vi "training_node.vi"() -> ()   [LabVIEW 2018]
uses:
  <vilib>/Utility/xml.llb/Read From XML File(string).vi
  <vilib>/Utility/xml.llb/Write to XML File(string).vi
panel:
  in  "Training Data Folder":path
  in  "Initialize Weights?":bool
  in  "Weights XML\n(Select Existing File or Name a New File)":path
  in  "Learning Parameter":dbl
  in  "Expected Output":dbl[](array[numeric])
  out "Output":dbl[](array[numeric])
  # "Neural Network Training Node"
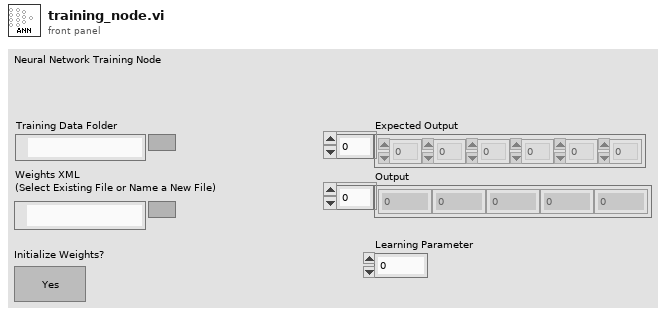
[diagram p1: front panel]
types:
  T1 = cluster{cluster{dbl[][], dbl[][], dbl[][]}, cluster{dbl[], dbl[], dbl[]}}
  T2 = enum16{"open", "replace", "create", "open or create", "replace or create", "replace or create with confirmation"}
  T3 = cluster{"Matrix Product":dbl[], "Matrix Product":dbl[], dbl[]}
  T4 = cluster{cluster{"Updated Weights":dbl[][], "Updated Weights":dbl[][], "Updated Weights":dbl[][]}, cluster{"Updated Biases":dbl[], "Updated Biases":dbl[], "Updated Biases":dbl[]}}
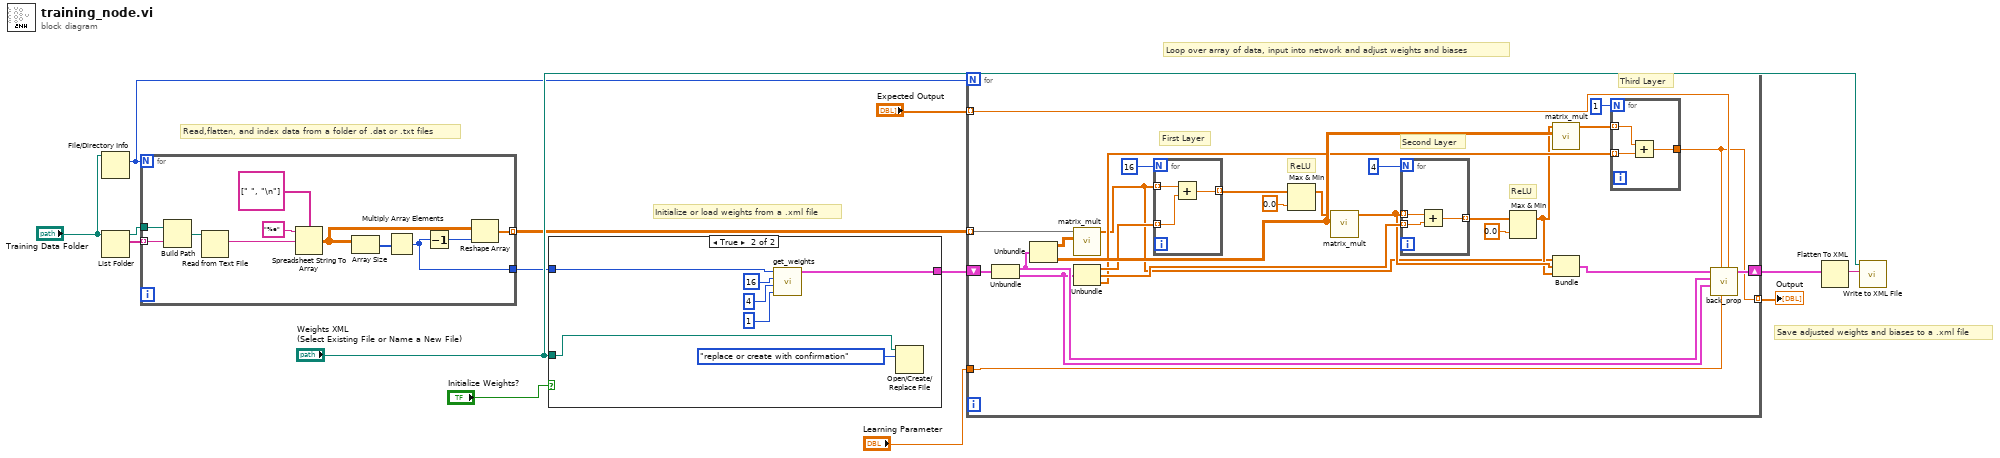
[diagram p0: block diagram]
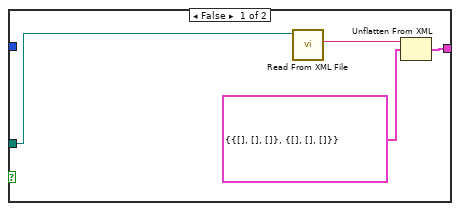
[diagram p2: hidden frame]
diagram:
  # "Save adjusted weights and biases to a .xml file"
  # "Loop over array of data, input into network and adjust weights and biases"
  # "Initialize or load weights from a .xml file"
  # "Read,flatten, and index data from a folder of .dat or .txt files"
  n1 = File/Directory Info(path="Training Data Folder") -> (size=w2:i64)  [unwired: 1 in, 6 out]
  n2 = List Folder(path="Training Data Folder") -> (path out=w6:path, filenames=w7:string[])  [unwired: 3 in, 2 out]
  n3 = for {
    N: w2 -> [_]
    tunnel: w7 -> [w25] mode=indexing
    tunnel: w6 -> [w24]
    tunnel: [w19] -> w4 mode=indexing
    tunnel: [w15] -> w1
    n4 = Build Path(base path=w24, name or relative path=w25) -> (appended path=w18:path)
    n5 = Read from Text File(file (use dialog)=w18) -> (text=w22:string)  [unwired: 3 in, 3 out]
    n6 = Spreadsheet String To Array(delimiter (Tab)=string[] [" ", "\n"], format string="%e", spreadsheet string=w22) -> (array=w17:dbl[][])  [unwired: 1 in]
    n7 = Array Size(array=w17) -> (size(s)=w16:i32[])
    n8 = Multiply Array Elements(1:w16) -> (0:w15:i32)
    n9 = Decrement(x=w15) -> (x-1=w20:i32)
    n10 = Reshape Array(w17, w20) -> (w19:dbl[])
  }
  n11 = case shown="True" "Initialize Weights?" {
    tunnel: "Weights XML\n(Select Existing File or Name a New File)" -> [w28 w33]
    tunnel: [w26 w31] -> w9
    tunnel: w1 -> [_ w30]
    frame False {
      n12 = call-poly <vilib>:"Read From XML File.vi"("XML File Path"=w28) -> ("XML Elements"=w29:string)  [unwired: 8 in, 2 out]
      n13 = Unflatten From XML(xml string=w29, type=T1 {{[], [], []}, {[], [], []}}) -> (value=w26:T1)  [unwired: 1 in, 1 out]
    }
    frame True {
      n14 = call "get_weights.vi"("Output Size"=1, "2H Size"=4, "1H Size"=16, "Input Size"=w30) -> ("Weights & Biases"=w31:T1)  [unwired: 7 in]
      n15 = Open/Create/Replace File(file path (use dialog)=w33, operation (0:open)=T2."replace or create with confirmation") -> ()  [unwired: 4 in, 3 out]
    }
  }
  n16 = for {
    N: w2 -> [_]
    tunnel: "Expected Output" -> [w44] mode=indexing
    tunnel: "Learning Parameter" -> [w43]
    shift-right: [w42] -> w8
    shift-left: w9 -> [w49]
    tunnel: w4 -> [w40] mode=indexing
    tunnel: [w37] -> w3 mode=indexing
    # "Third Layer"
    # "Second Layer"
    # "First Layer"
    # "ReLU"
    # "ReLU"
    n17 = Unbundle(w49) -> (w45:cluster{dbl[][], dbl[][], dbl[][]}, w41:cluster{dbl[], dbl[], dbl[]})
    n18 = Unbundle(w45) -> (w54:dbl[][], w53:dbl[][])  [unwired: 1 out]
    n19 = call "matrix_mult.vi"("Weights"=w54, "Input Array"=w40) -> ("Matrix Product"=w39:dbl[])  [unwired: 9 in]
    n20 = Unbundle(w41) -> (w52:dbl[], w51:dbl[], w50:dbl[])
    n21 = for {
      N: 16 -> [_]
      tunnel: [w71] -> w62 mode=indexing
      tunnel: w39 -> [w70] mode=indexing
      tunnel: w52 -> [w69] mode=indexing
      n22 = Add(x=w70, y=w69) -> (x+y=w71:dbl)
    }
    n23 = Max & Min(x=w62, y=0.0) -> (max(x,y)=w48:dbl[])  [unwired: 1 out]
    n24 = call "matrix_mult.vi"("Weights"=w53, "Input Array"=w48) -> ("Matrix Product"=w47:dbl[])  [unwired: 9 in]
    n25 = for {
      N: 4 -> [_]
      tunnel: [w68] -> w56 mode=indexing
      tunnel: w47 -> [w67] mode=indexing
      tunnel: w51 -> [w66] mode=indexing
      n26 = Add(x=w67, y=w66) -> (x+y=w68:dbl)
    }
    n27 = Max & Min(x=w56, y=0.0) -> (max(x,y)=w46:dbl[])  [unwired: 1 out]
    n28 = call "matrix_mult.vi"("Weights"=w53, "Input Array"=w46) -> ("Matrix Product"=w55:dbl[])  [unwired: 9 in]
    n29 = Bundle("Matrix Product"=w39, "Matrix Product"=w47, w46) -> (w38:T3)  [unwired: 1 in]
    n30 = for {
      N: 1 -> [_]
      tunnel: [w65] -> w37
      tunnel: w55 -> [w64] mode=indexing
      tunnel: w50 -> [w63] mode=indexing
      n31 = Add(x=w64, y=w63) -> (x+y=w65:dbl)
    }
    n32 = call "back_prop.vi"("Expected Output"=w44, "Learning Parameter"=w43, "Output"=w37, "Biases"=w41, "Weights"=w45, "Data Output"=w38) -> ("output cluster"=w42:T4)  [unwired: 5 in]
  }
  "Output" <- w3
  n33 = Flatten To XML(anything=w8) -> (xml string=w11:string)
  n34 = call-poly <vilib>:"Write to XML File.vi"("XML Input"=w11, "XML File Path"="Weights XML\n(Select Existing File or Name a New File)") -> ()  [unwired: 7 in, 3 out]
